vi "Q.Pong.vi"(8 "Error In":errorcluster, 11 "Data In":variant) -> (0 "Error Out":errorcluster)   [LabVIEW 2024, in "EQMF.lvlib" / "Queue Utils.lvlib"]
doc: "This VI enqueues an element to the Queue.\nIf the 'Q Name' input is not empty then it obtains the queue by name.\n If a queue is ontained by name and this queue does nto already exits, an error is generated.\nIf the 'Q Name' input is empty then it uses the 'Q In' for obtaining the queue.\n\nBy default the 'Top of Q' input is FALSE to put this element on bottom of the queue.\nSet 'Top of Q' to TRUE to enqueue this command at the top of the queue."
uses:
  Queue Utils.lvlib
  Q.Element.ctl
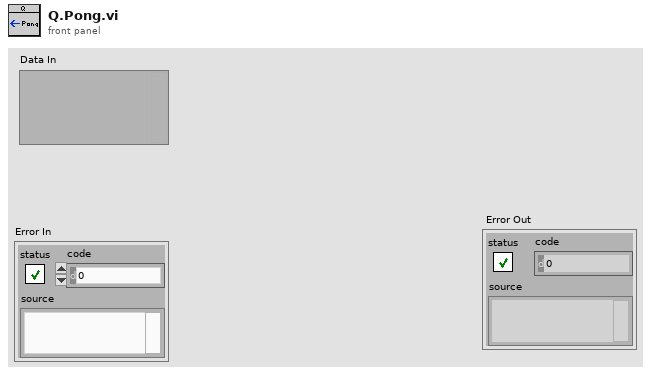
[diagram p1: front panel]
types:
  T1 = typedef "EQMF.lvlib/Queue Utils.lvlib/Q.Element.ctl" = cluster{"Cmd":string, "Sub":string, "Data1":variant, "Data2":variant}
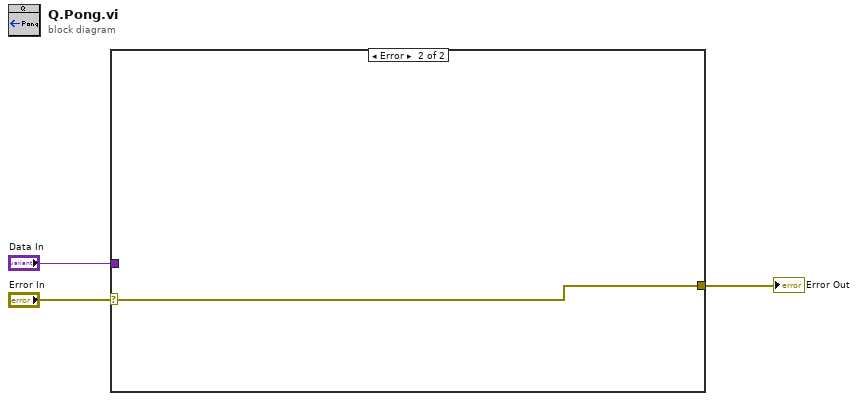
[diagram p0: block diagram]
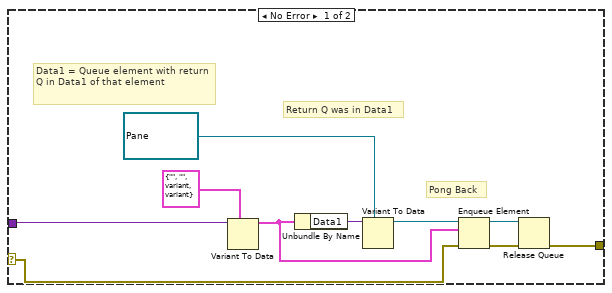
[diagram p2: hidden frame]
diagram:
  n1 = case shown="Error" "Error In" {
    selector: "Error In" -> [w8 w14]
    tunnel: [w4 w14] -> w3
    tunnel: "Data In" -> [w13 _]
    frame No Error {
      # "Data1 = Queue element with return Q in Data1 of that element"
      # "Pong Back"
      # "Return Q was in Data1"
      n2 = Variant To Data(type=T1 {"Cmd"="", "Sub"="", "Data1"=variant, "Data2"=variant}, Variant=w13) -> (data=w9:T1)  [unwired: 1 in, 1 out]
      n3 = Unbundle By Name(w9) -> ("Data1"=w12:variant)
      n4 = Variant To Data(type=refnum<queue> refnum ("queue out"), Variant=w12) -> (data=w10:refnum<queue>)  [unwired: 1 in, 1 out]
      n5 = Enqueue Element(queue=w10, element=w9, error in (no error)=w8) -> (queue out=w5:refnum<queue>, error out=w6:errorcluster)  [unwired: 1 in, 1 out]
      n6 = Release Queue(queue=w5, error in (no error)=w6) -> (error out=w4:errorcluster)  [unwired: 1 in, 2 out]
    }
    frame Error {
    }
  }
  "Error Out" <- w3
